vi "Dielectric Material Properties GAP.vi"(8 "Dielectric Thickness Total":dbl, 9 "Energy (Heat; I^2R)":dbl, 11 "NS Base Area":dbl) -> (0 "Dielectric Specfic Heat Capacity":dbl, 1 "Mass Dielectric":dbl, 2 "Dielectric Density":dbl, 3 "Volume Dielectric":dbl, 4 "Delta Temp Change \nDielectric":dbl, 5 "Dielectric Thickness  out":dbl)   [LabVIEW 2020]
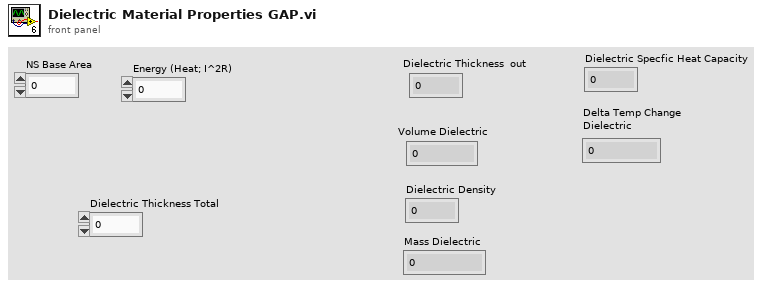
[diagram p1: front panel]
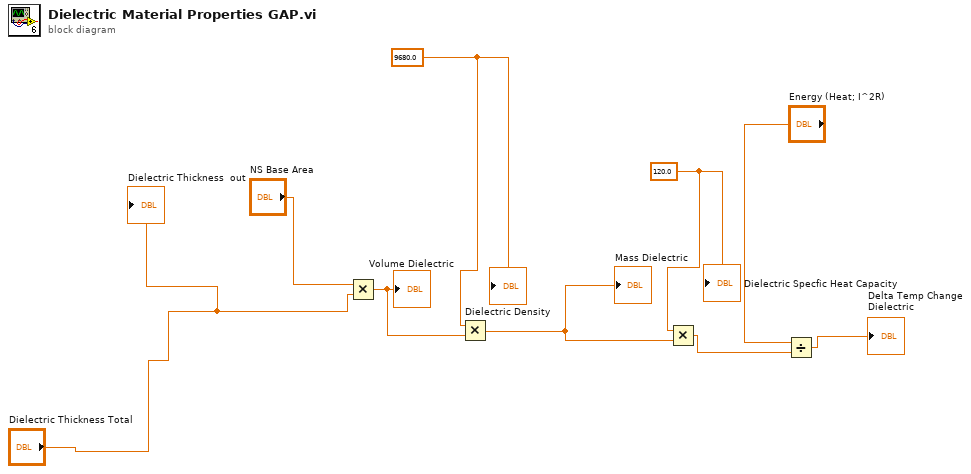
[diagram p0: block diagram]
diagram:
  w2 = 120.0 ("Silicon Specfic Heat Capacity 8")
  w3 = 9680.0 ("Silicon Density 8")
  n1 = Multiply(x="NS Base Area", y="Dielectric Thickness Total") -> (x*y=w4:dbl)
  "Volume Dielectric" <- w4
  n2 = Multiply(x=w3, y=w4) -> (x*y=w9:dbl)
  "Mass Dielectric" <- w9
  n3 = Multiply(x=w2, y=w9) -> (x*y=w8:dbl)
  n4 = Divide(x="Energy (Heat; I^2R)", y=w8) -> (x/y=→"Delta Temp Change \nDielectric":dbl)
  "Dielectric Thickness  out" <- "Dielectric Thickness Total"
  "Dielectric Density" <- w3
  "Dielectric Specfic Heat Capacity" <- w2
